vi "Error Write Status.vi"(8 "error in":errorcluster, 10 "Error STS":i32, 11 "Climate Chamber in":refnum<class "Climate Chamber.lvclass">) -> (0 "error out":errorcluster, 3 "Climate Chamber out":refnum<class "Climate Chamber.lvclass">)   [LabVIEW 2023, in "Climate Chamber.lvclass"]
uses:
  Climate Chamber.lvclass
  Climate Chamber.lvclass/Climate Chamber.ctl
  Low Level Capabilities/Error/Error.lvclass
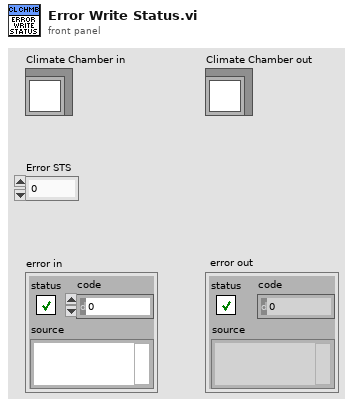
[diagram p1: front panel]
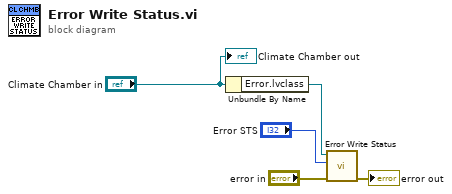
[diagram p0: block diagram]
diagram:
  n1 = Unbundle By Name("Climate Chamber in") -> ("Error.lvclass"=w5:refnum<class "Error.lvclass">)
  n2 = call-dynamic "Error Write Status.vi"("error in"="error in", "Error STS"="Error STS", "Error in"=w5) -> ("error out"=→"error out":errorcluster)  [unwired: 7 in, 1 out]
  "Climate Chamber out" <- "Climate Chamber in"
